vi "nodeInfo.get library version.vi"() -> (0 "nameAndVersion":string)   [LabVIEW 2012, in "LVNodeInfo.lvlib"]
doc: "get name and version of this library as a string"
uses:
  LVNodeInfo.lvlib
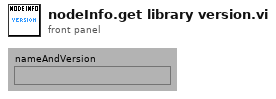
[diagram p1: front panel]
types:
  T1 = cluster{"Major":u16, "Minor":u16, "Fix":u16, "Build":u16}
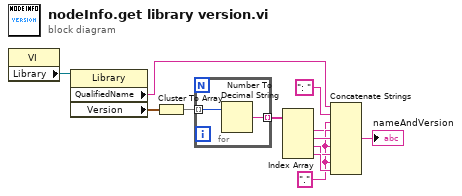
[diagram p0: block diagram]
diagram:
  w9 = "." ("string")
  n1 = property class="VI"() -> ("Library"=w2:refnum<vi>)  [unwired: 2 in, 2 out]
  n2 = property class="Library"(reference=w2) -> ("QualifiedName"=w6:string, "Version"=w3:T1)  [unwired: 1 in, 2 out]
  n3 = Cluster To Array(cluster=w3) -> (array=w4:u16[])
  n4 = for {
    tunnel: w4 -> [w14] mode=indexing
    tunnel: [w13] -> w5 mode=indexing
    n5 = Number To Decimal String(number=w14) -> (decimal integer string=w13:string)  [unwired: 1 in]
  }
  n6 = Index Array(array=w5) -> (element #1=w8:string, element #2=w10:string, element #3=w11:string, element #4=w12:string)  [unwired: 4 in]
  n7 = Concatenate Strings(w6, ": " ("string"), w8, w9, w10, w9, w11, w9, w12) -> (→"nameAndVersion":string)
